vi "queryHardpointActuatorStatus.vi"(8 "error in (no error)":errorcluster, 9 "TriggerIRQ":bool, 10 "WaitForTrigger":bool, 11 "Model in":refnum<class "Model.lvclass">) -> (0 "error out":errorcluster, 3 "Model out":refnum<class "Model.lvclass">)   [LabVIEW 2016, in "Model.lvclass"]
uses:
  Model.lvclass
  Model.lvclass/Model.ctl
  ILCCommunications/ILCCommunications.lvclass
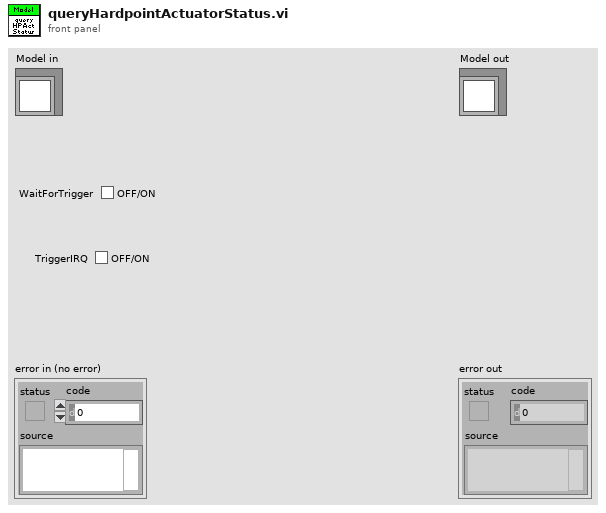
[diagram p1: front panel]
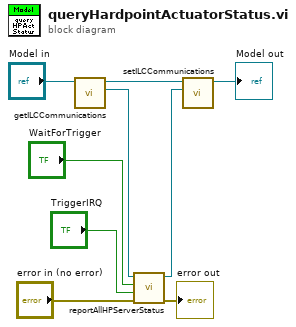
[diagram p0: block diagram]
diagram:
  n1 = call "getILCCommunications.vi"("Model in"="Model in") -> ("ILCCommunications"=w6:refnum<class "ILCCommunications.lvclass">, "Model out"=w8:refnum<class "Model.lvclass">)  [unwired: 9 in]
  n2 = call "reportAllHPServerStatus.vi"("error in (no error)"="error in (no error)", "TriggerIRQ"="TriggerIRQ", "WaitForTrigger"="WaitForTrigger", "ILCCommunications in"=w6) -> ("error out"=→"error out":errorcluster, "ILCCommunications out"=w5:refnum<class "ILCCommunications.lvclass">)  [unwired: 6 in]
  n3 = call "setILCCommunications.vi"("ILCCommunications"=w5, "Model in"=w8) -> ("Model out"=→"Model out":refnum<class "Model.lvclass">)  [unwired: 9 in]
